vi "angle_to_setpoint.vi"() -> ()   [LabVIEW 2020]
uses:
  <vilib>/Math Plots/2D Math Plots/2D Compass/2D Compass XCtrl/2D Compass.xctl
  <vilib>/Analysis/coordinate.llb/Angle Units.ctl
  <vilib>/Analysis/coordinate.llb/Angle Range (Degree).ctl
  <vilib>/Analysis/coordinate.llb/Wrap Angle (scalar).vi
  <vilib>/Math Plots/2D Math Plots/2D Compass/2D Compass Datatype/Public/Plot Helper (Vector).vi
  <vilib>/Math Plots/2D Math Plots/2D Compass/2D Compass Datatype/2D Compass Datatype.lvclass
  <vilib>/Analysis/NI_AAL_Angle.lvlib
panel:
  out "Theta":dbl
  out "Min":dbl
  out "Max":dbl
  out "2D Compass":refnum<class "2D Plot Datatype.lvclass">[](xcontrol)
  in  "Desired":dbl
  in  "Current":dbl
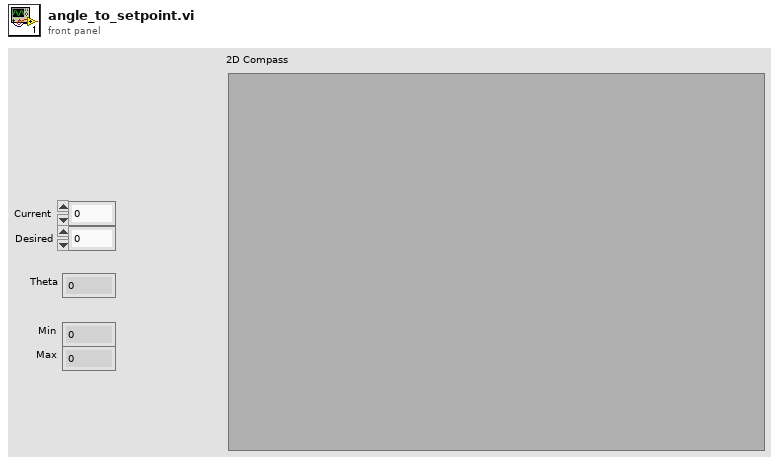
[diagram p1: front panel]
types:
  T1 = typedef "NI_AAL_Angle.lvlib/Angle Range (Degree).ctl" = u16
  T2 = typedef "NI_AAL_Angle.lvlib/Angle Units.ctl" = i32
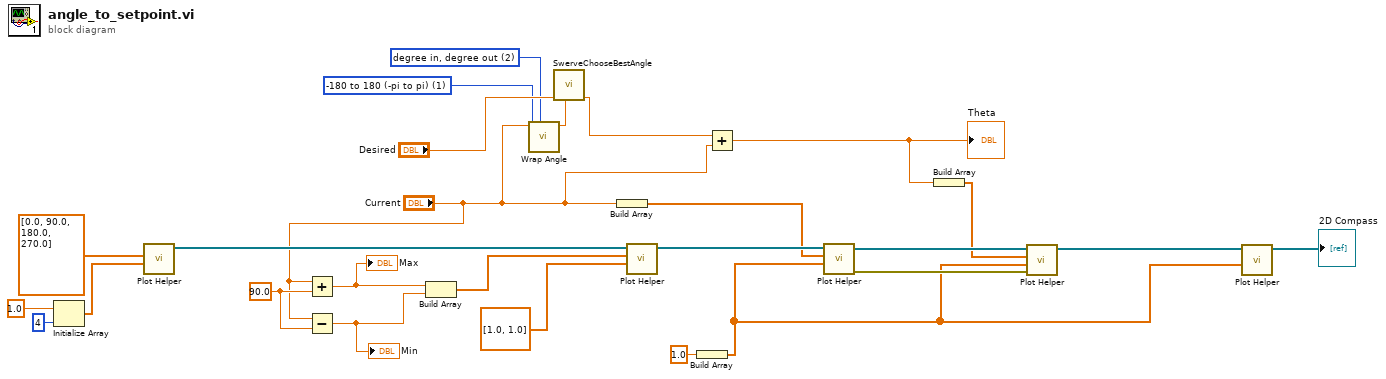
[diagram p0: block diagram]
diagram:
  w2 = T1 1 items=["none", "-180 to 180 (-pi to pi)", "0 to 360 (0 to 2pi)"] ("angle range")
  w4 = T2 2 items=["radian in, radian out", "radian in, degree out", "degree in, degree out", "degree in, radian out"] ("angle units")
  w16 = 90.0 ("y")
  n1 = Initialize Array(1.0 ("element"), 4 ("dimension size")) -> (w22:dbl[])
  n2 = call-poly <vilib>:"Plot Helper.vi"("radius vector"=w22, "theta vector"=dbl[] [0.0, 90.0, 180.0, 270.0]) -> ("2D Plot Class Obj Array out"=w23:refnum<class "2D Plot Datatype.lvclass">[])  [unwired: 2 in, 7 out]
  n3 = Add(x="Current", y=w16) -> (x+y=w10:dbl)
  "Max" <- w10
  n4 = Subtract(x="Current", y=w16) -> (x-y=w11:dbl)
  "Min" <- w11
  n5 = Build Array(w10, w11) -> (w17:dbl[])
  n6 = call-poly <vilib>:"Wrap Angle.vi"("angle units"=w4, "angle range"=w2, "angle in"="Current") -> ("angle out"=w3:dbl)  [unwired: 7 in, 1 out]
  n7 = call "SwerveChooseBestAngle.vi"("Current Angle"=w3, "Target Angle"="Desired") -> ("Setpoint Angle"=w5:dbl)  [unwired: 8 in, 1 out]
  n8 = Build Array("Current") -> (w19:dbl[])
  n9 = call-poly <vilib>:"Plot Helper.vi"("radius vector"=dbl[] [1.0, 1.0], "theta vector"=w17, "2D Plot Class Obj Array in"=w23) -> ("2D Plot Class Obj Array out"=w21:refnum<class "2D Plot Datatype.lvclass">[])  [unwired: 1 in, 7 out]
  n10 = Build Array(1.0 ("element")) -> (w8:dbl[])
  n11 = Add(x=w5, y="Current") -> (x+y=w6:dbl)
  "Theta" <- w6
  n12 = call-poly <vilib>:"Plot Helper.vi"("radius vector"=w8, "theta vector"=w19, "2D Plot Class Obj Array in"=w21) -> ("error out"=w14:errorcluster, "2D Plot Class Obj Array out"=w15:refnum<class "2D Plot Datatype.lvclass">[])  [unwired: 1 in, 6 out]
  n13 = Build Array(w6) -> (w9:dbl[])
  n14 = call-poly <vilib>:"Plot Helper.vi"("error in (no error)"=w14, "radius vector"=w8, "theta vector"=w9, "2D Plot Class Obj Array in"=w15) -> ("2D Plot Class Obj Array out"=w13:refnum<class "2D Plot Datatype.lvclass">[])  [unwired: 7 out]
  n15 = call-poly <vilib>:"Plot Helper.vi"("radius vector"=w8, "2D Plot Class Obj Array in"=w13) -> ("2D Plot Class Obj Array out"=→"2D Compass":refnum<class "2D Plot Datatype.lvclass">[])  [unwired: 2 in, 7 out]
